vi "WriteAccess.vi"(8 "error in (no error)":errorcluster, 10 "Access":T1, 11 "BaseAccessorScripter in":refnum<class "BaseAccessorScripter.lvclass">) -> (0 "error out":errorcluster, 3 "BaseAccessorScripter out":refnum<class "BaseAccessorScripter.lvclass">)   [LabVIEW 2021, in "MemberVICreation.lvlib" / "BaseAccessorScripter.lvclass"]
uses:
  <resource>/Framework/Providers/LVClassLibrary/NewAccessors/BaseAccessorScripter/BaseAccessorScripter.lvclass
  <resource>/Framework/Providers/LVClassLibrary/NewAccessors/CLSUIP_Access.ctl
  <resource>/Framework/Providers/LVClassLibrary/NewAccessors/BaseAccessorScripter/BaseAccessorScripter.lvclass/BaseAccessorScripter.ctl
  <resource>/Framework/Providers/LVClassLibrary/NewAccessors/MemberVICreation.lvlib
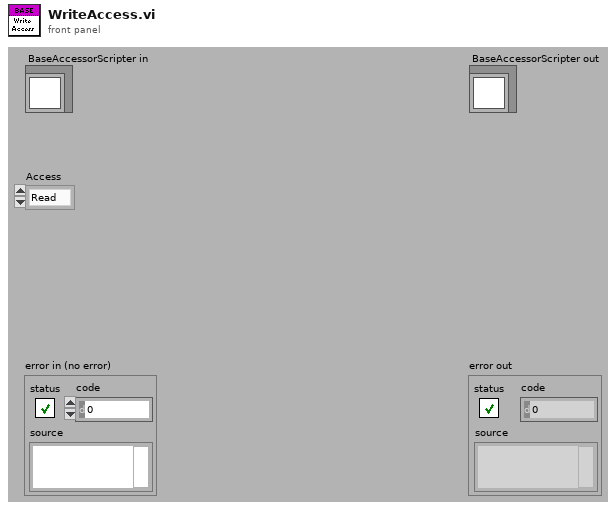
[diagram p1: front panel]
types:
  T1 = typedef "MemberVICreation.lvlib/CLSUIP_Access.ctl" = enum16{"Read", "Write", "R/W"}
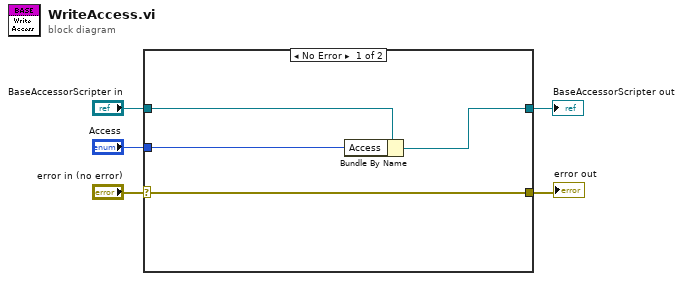
[diagram p0: block diagram]
diagram:
  n1 = case shown="No Error" "error in (no error)" {
    selector: "error in (no error)" -> [w9 w11]
    tunnel: [w9 w11] -> w4
    tunnel: [w7 w10] -> w2
    tunnel: "BaseAccessorScripter in" -> [w8 w10]
    tunnel: "Access" -> [w6 _]
    frame No Error {
      n2 = Bundle By Name(cluster=w8, "Access"=w6) -> (w7:refnum<class "BaseAccessorScripter.lvclass">)
    }
    frame Error {
    }
  }
  "error out" <- w4
  "BaseAccessorScripter out" <- w2
